vi "Sigma_SendCmd.vi"(8 "error in (no error)":errorcluster, 9 "String to Receive":string="OK", 10 "String to Send":string, 11 "VISA resource name":refnum<visa-resource-name>) -> (0 "error out":errorcluster, 1 "String Received":string, 2 "OK Done":bool, 3 "VISA resource name out":refnum<visa-resource-name>)   [LabVIEW 2018]
panel:
  out "연결된 문자열":string
  # "Port Number 0=COM1"
  # "Send the 'String to Send' to the Stage Controller and wait for the 'String to Receive'.\nAn Error occurs when received a different string or timed out."
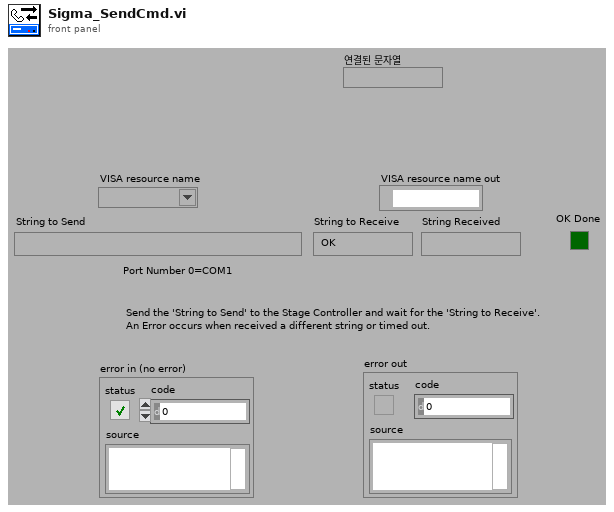
[diagram p1: front panel]
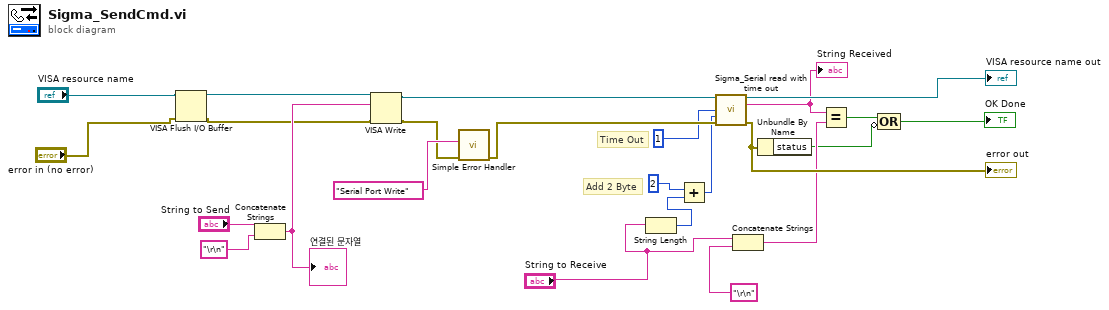
[diagram p0: block diagram]
diagram:
  # "Time Out"
  # "Add 2 Byte"
  n1 = VISA Flush I/O Buffer(VISA resource name="VISA resource name", error in (no error)="error in (no error)") -> (VISA resource name out=w1:refnum<visa-resource-name>, error out=w2:errorcluster)  [unwired: 1 in]
  n2 = Concatenate Strings("String to Send", "\r\n") -> (w15:string)
  "연결된 문자열" <- w15
  n3 = VISA Write(VISA resource name=w1, write buffer=w15, error in (no error)=w2) -> (VISA resource name out=w18:refnum<visa-resource-name>, error out=w17:errorcluster)  [unwired: 1 out]
  n4 = call <vilib>:"Simple Error Handler.vi"("error source (\" \")"="Serial Port Write", "error in (no error)"=w17) -> ("error out"=w22:errorcluster)  [unwired: 2 in, 5 out]
  n5 = String Length(string="String to Receive") -> (length=w14:i32)
  n6 = Add(x=2, y=w14) -> (x+y=w8:i32)
  n7 = call "Sigma_Serial read with time out.vi"("VISA resource name"=w18, "Time out"=1, "Byte to read"=w8, "error in (no error)"=w22) -> ("VISA resource name out"=→"VISA resource name out":refnum<visa-resource-name>, "read buffer"=w5:string, "error out"=w21:errorcluster)  [unwired: 8 in, 1 out]
  "error out" <- w21
  "String Received" <- w5
  n8 = Concatenate Strings("String to Receive", "\r\n") -> (w10:string)
  n9 = Unbundle By Name(w21) -> ("status"=w6:bool)
  n10 = Equal?(x=w5, y=w10) -> (x = y?=w7:bool)
  n11 = Compound Arithmetic op=OR(w7, invert w6) -> (→"OK Done":bool)
